vi "IStageDyPos.vi"(0 "PRIORLib.IStageIn":refnum<k7>, 1 "PRIORLib.IScanIn":refnum<k7>) -> (2 "PRIORLib.IStageOut":refnum<k7>, 3 "PRIORLib.IScanOut":refnum<k7>, 4 "XPos":dbl, 5 "YPos":dbl)   [LabVIEW 2016]
uses:
  Globals.vi
panel:
  out "IScanError":errorcluster
  out "IStageError":errorcluster
  out "Return":u32
  out "Moving":bool
  # "This SubVi gets the stage position every 100 ms. while\nthe stage is moving, then returns the final stage location\nafter the stage stops."
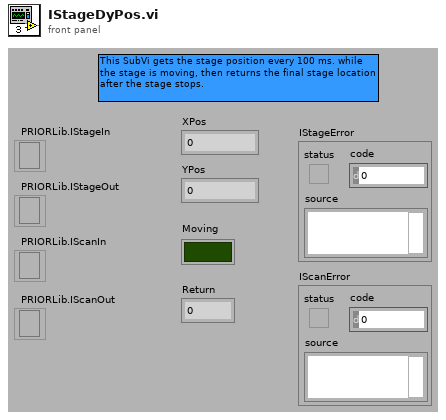
[diagram p1: front panel]
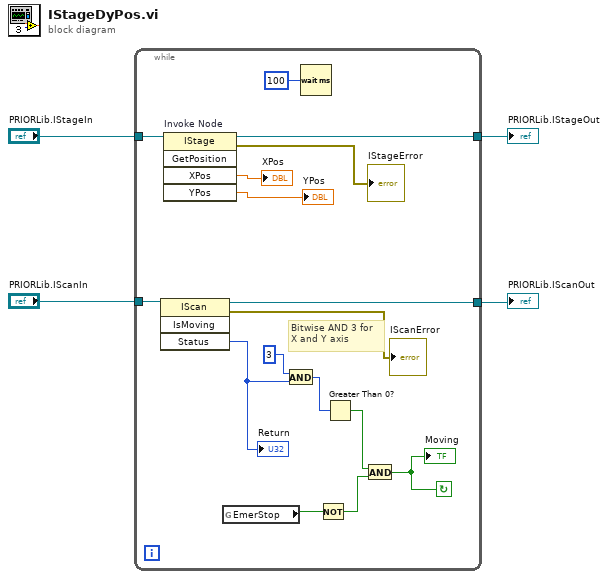
[diagram p0: block diagram]
diagram:
  n1 = while {
    tunnel: "PRIORLib.IStageIn" -> [w20]
    tunnel: [w19] -> w3
    tunnel: "PRIORLib.IScanIn" -> [w16]
    tunnel: [w15] -> w1
    stop <- w7 continue-if-true
    # "Bitwise AND 3 for\nX and Y axis"
    n2 = invoke class="IScan" method="IsMoving"(reference=w16) -> (reference out=w15:refnum<k7>, error out=→"IScanError":errorcluster, "Status"=w10:i32)  [unwired: 3 in, 1 out]
    "Return" <- w10
    n3 = invoke on="Invoke Node" class="IStage" method="GetPosition"(reference=w20) -> (reference out=w19:refnum<k7>, error out=→"IStageError":errorcluster, "XPos"=→"XPos":dbl, "YPos"=→"YPos":dbl)  [unwired: 4 in, 1 out]
    n4 = global read "Globals.vi" "EmerStop"() -> (w6:bool)
    n5 = And(x=3, y=w10) -> (x .and. y?=w9:i32)
    n6 = Wait (ms)(milliseconds to wait=u32 100) -> ()  [unwired: 1 out]
    n7 = Not(x=w6) -> (.not. x?=w5:bool)
    n8 = Greater Than 0?(x=w9) -> (x > 0?=w8:bool)
    n9 = And(x=w8, y=w5) -> (x .and. y?=w7:bool)
    "Moving" <- w7
  }
  "PRIORLib.IStageOut" <- w3
  "PRIORLib.IScanOut" <- w1
